vi "Pracownia6.vi"() -> ()   [LabVIEW 2019]
uses:
  Pracowania_6_global.vi
panel:
  out "Liczba binarnie":bool[](array[boolean])
  in  "Zero":bool
  in  "Liczba":u8
  in  "stop":bool
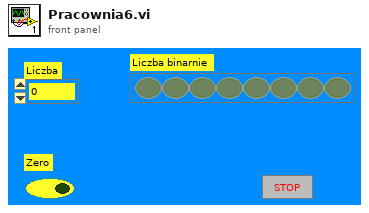
[diagram p1: front panel]
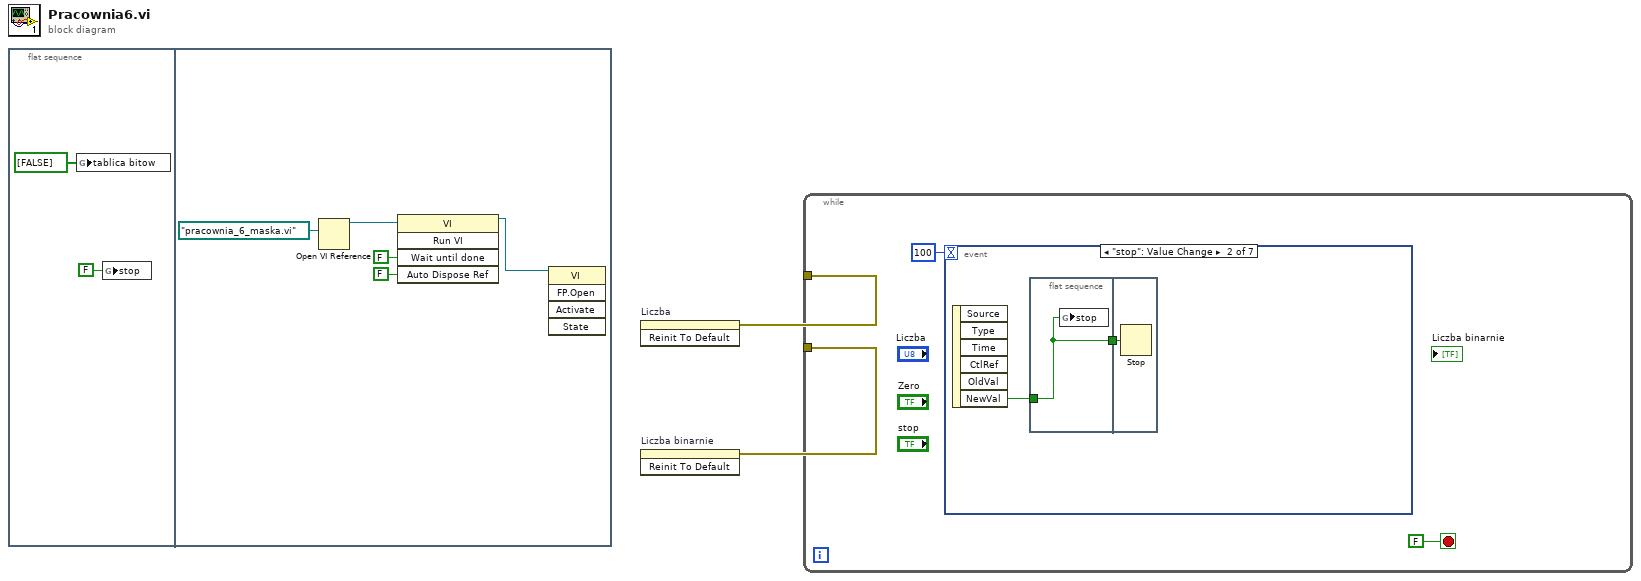
[diagram p0: block diagram]
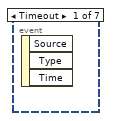
[diagram p2: hidden frame]
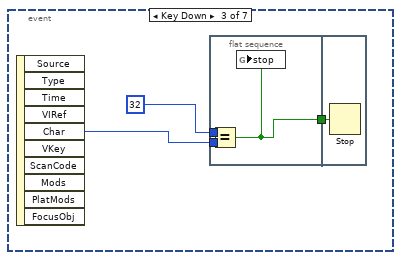
[diagram p3: hidden frame]
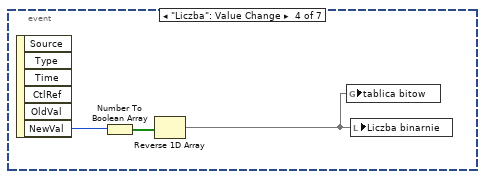
[diagram p4: hidden frame]
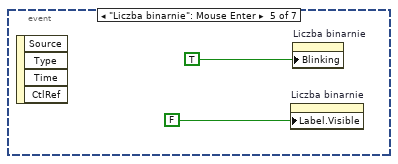
[diagram p5: hidden frame]
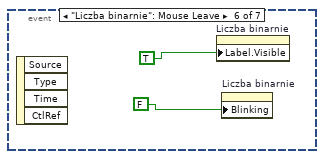
[diagram p6: hidden frame]
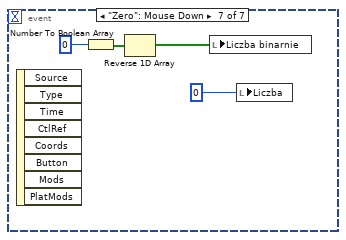
[diagram p7: hidden frame]
diagram:
  n1 = flat-sequence {
    frame #0 {
      n2 = global write "Pracowania_6_global.vi" "tablica bitow"(bool[] [FALSE] ("tablica bitow")) -> ()
      n3 = global write "Pracowania_6_global.vi" "stop"(FALSE ("stop")) -> ()
    }
    frame #1 {
      n4 = Open VI Reference(vi path=path "pracownia_6_maska.vi") -> (vi reference=w9:refnum<vi>)  [unwired: 5 in, 1 out]
      n5 = invoke class="VI" method="Run VI"(reference=w9, "Wait until done"=FALSE ("Wait Until Done"), "Auto Dispose Ref"=FALSE ("Auto Dispose Reference")) -> (reference out=w8:refnum<vi>)  [unwired: 2 in, 4 out]
      n6 = invoke class="VI" method="FP.Open"(reference=w8) -> ()  [unwired: 4 in, 5 out]
    }
  }
  n7 = invoke on="Liczba" class="DigNum (strict)" method="Reinit To Default"() -> (error out=w1:errorcluster)  [unwired: 3 in, 2 out]
  n8 = invoke on="Liczba binarnie" class="Arr (strict)" method="Reinit To Default"() -> (error out=w2:errorcluster)  [unwired: 3 in, 2 out]
  n9 = while {
    tunnel: w2 -> [_]
    tunnel: w1 -> [_]
    stop <- FALSE stop-if-true
    n10 = event shown="[1] \"stop\": Value Change" {
      selector: _ -> [_ _ _ _ _ _ _]
      dyn-events: _ -> [_ _ _ _ _ _ _]
      timeout: 100 -> [_ _ _ _ _ _ _]
      event Timeout {
        n11 = event-data() -> ()  [unwired: 1 in, 3 out]
      }
      event "stop": Value Change {
        n12 = event-data() -> ("NewVal"=w13:bool)  [unwired: 1 in, 5 out]
        n13 = flat-sequence {
          tunnel: w13 -> [w14]
          tunnel: [w14] -> w12
          tunnel: w12 -> [w15]
          frame #0 {
            n14 = global write "Pracowania_6_global.vi" "stop"(w14) -> ()
          }
          frame #1 {
            n15 = Stop(stop? (T)=w15) -> ()
          }
        }
      }
      event Key Down {
        n16 = event-data() -> ("Char"=w18:i16)  [unwired: 1 in, 9 out]
        n17 = flat-sequence {
          tunnel: w18 -> [w21]
          tunnel: 32 -> [w20]
          tunnel: [w19] -> w16
          tunnel: w16 -> [w22]
          frame #0 {
            n18 = Equal?(x=w20, y=w21) -> (x = y?=w19:bool)
            n19 = global write "Pracowania_6_global.vi" "stop"(w19) -> ()
          }
          frame #1 {
            n20 = Stop(stop? (T)=w22) -> ()
          }
        }
      }
      event "Liczba": Value Change {
        n21 = event-data() -> ("NewVal"=w25:u8)  [unwired: 1 in, 5 out]
        n22 = Number To Boolean Array(number=w25) -> (Boolean array=w24:bool[])
        n23 = Reverse 1D Array(array=w24) -> (reversed array=w23:bool[])
        n24 = global write "Pracowania_6_global.vi" "tablica bitow"(w23) -> ()
        n25 = local write "Liczba binarnie"(w23) -> ()
      }
      event "Liczba binarnie": Mouse Enter {
        n26 = event-data() -> ()  [unwired: 1 in, 4 out]
        n27 = property on="Liczba binarnie" class="Arr (strict)"("Label.Visible"=FALSE) -> ()  [unwired: 2 in, 2 out]
        n28 = property on="Liczba binarnie" class="Arr (strict)"("Blinking"=TRUE) -> ()  [unwired: 2 in, 2 out]
      }
      event "Liczba binarnie": Mouse Leave {
        n29 = event-data() -> ()  [unwired: 1 in, 4 out]
        n30 = property on="Liczba binarnie" class="Arr (strict)"("Label.Visible"=TRUE) -> ()  [unwired: 2 in, 2 out]
        n31 = property on="Liczba binarnie" class="Arr (strict)"("Blinking"=FALSE) -> ()  [unwired: 2 in, 2 out]
      }
      event "Zero": Mouse Down {
        n32 = event-data() -> ()  [unwired: 1 in, 8 out]
        n33 = Number To Boolean Array(number=u8 0) -> (Boolean array=w31:bool[])
        n34 = Reverse 1D Array(array=w31) -> (reversed array=w30:bool[])
        n35 = local write "Liczba binarnie"(w30) -> ()
        n36 = local write "Liczba"(u8 0 ("Liczba")) -> ()
      }
    }
  }
